vi "real_web_report.vi"(11 "httpRequestID":u32) -> (3 "httpRequestID out":u32)   [LabVIEW 2011]
uses:
  <vilib>/addons/database/Connection.llb/DB Tools Open Connec (String).vi
  databasePath.vi
  <vilib>/addons/database/Connection.llb/Conn Execute.vi
  <vilib>/addons/database/Recordset.llb/Rec Fetch Recordset Data (R).vi
  <vilib>/addons/database/Recordset.llb/Rec Destroy - Connection.vi
  <vilib>/addons/database/NI_Database_API.lvlib
  <vilib>/wsapi/NI_WebServices.lvlib
panel:
  out "error out":errorcluster
  out "error out 2":errorcluster
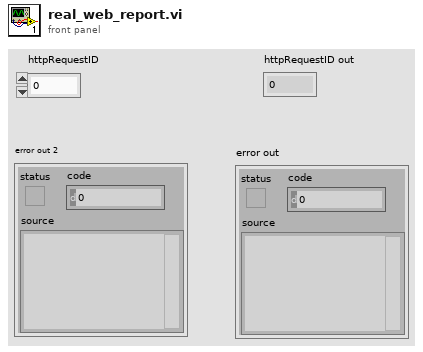
[diagram p1: front panel]
types:
  T1 = typedef "NI_Database_API.lvlib/Conn ObjectReference.ctl" = refnum<k1>
  T2 = typedef "NI_Database_API.lvlib/Rec ObjectReference.ctl" = refnum<k1>
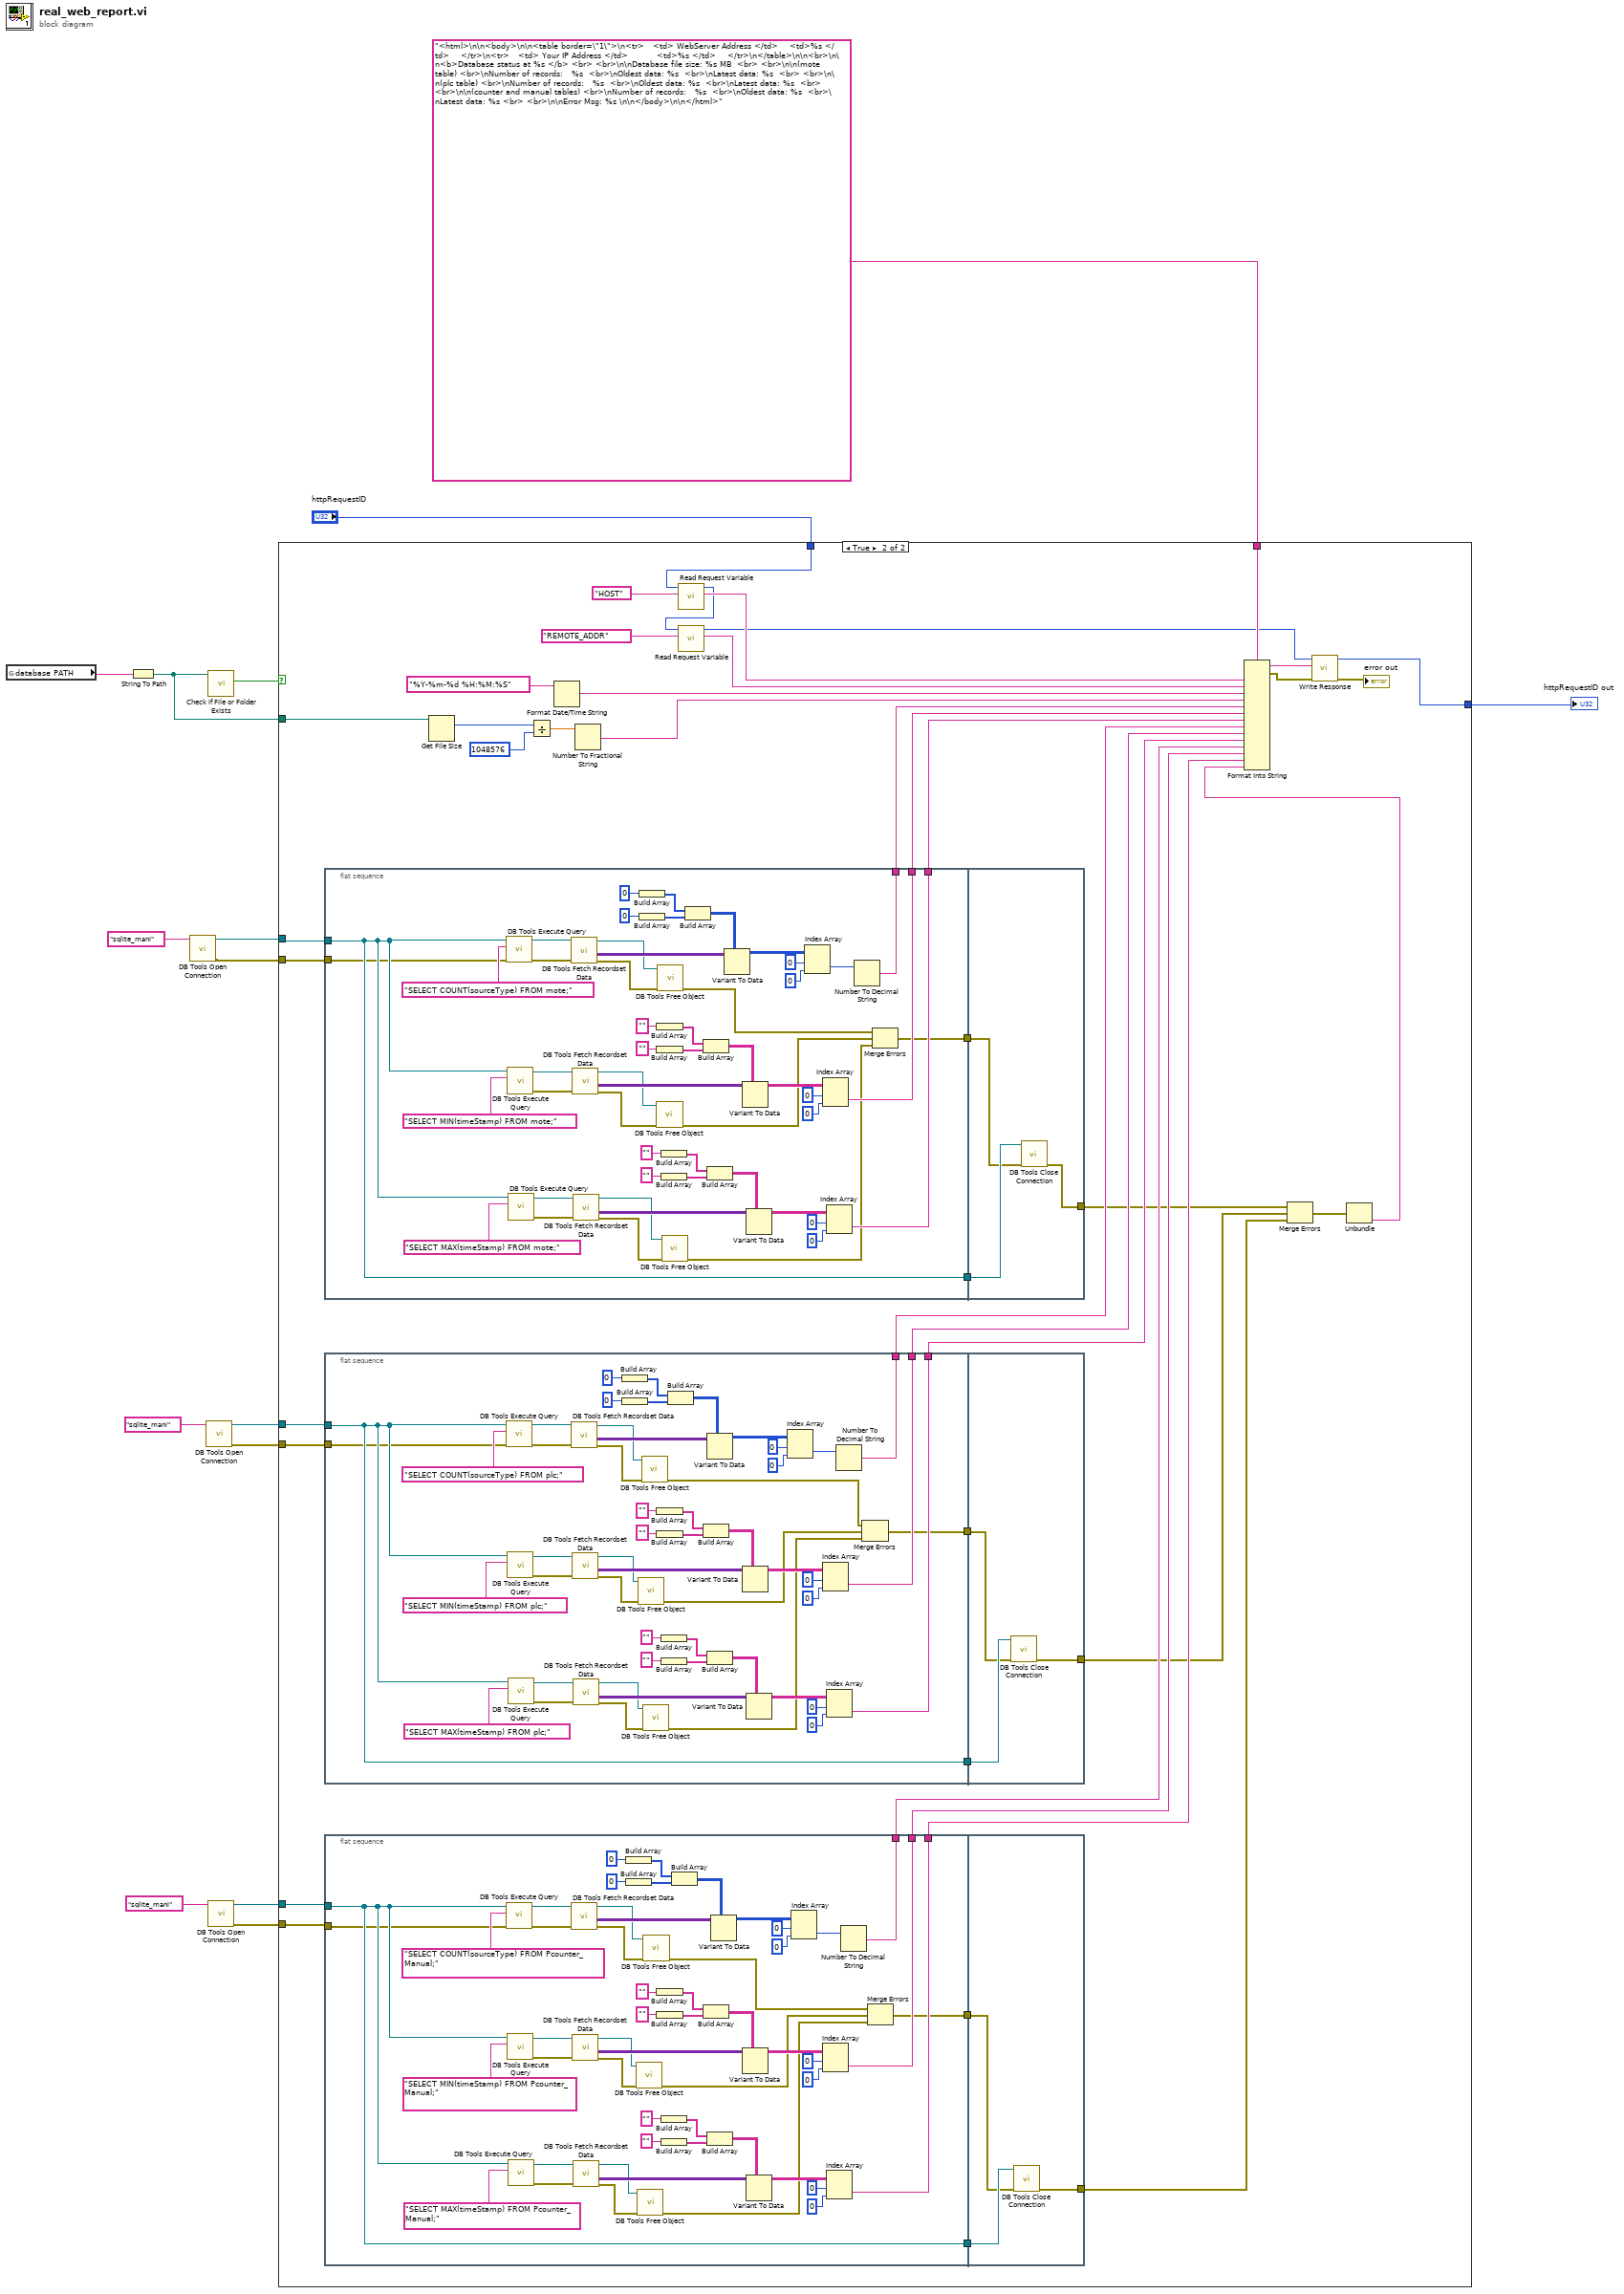
[diagram p0: block diagram]
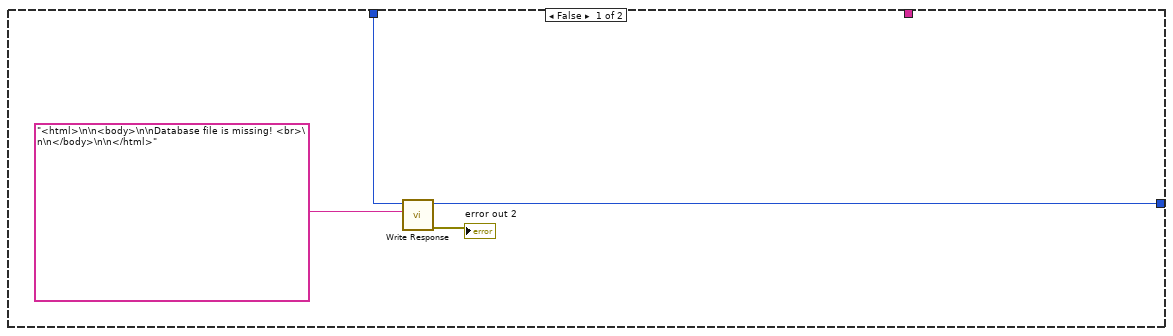
[diagram p2: hidden frame]
diagram:
  n1 = global read "databasePath.vi" "database PATH"() -> (w14:string)
  n2 = String To Path(string=w14) -> (path=w13:path)
  n3 = call-poly <vilib>:"DB Tools Open Connection.vi"("connection information"="sqlite_mani") -> ("error out"=w8:errorcluster, "connection reference"=w9:T1)  [unwired: 7 in]
  n4 = call-poly <vilib>:"DB Tools Open Connection.vi"("connection information"="sqlite_mani") -> ("error out"=w3:errorcluster, "connection reference"=w4:T1)  [unwired: 7 in]
  n5 = call <vilib>:"Check if File or Folder Exists.vi"("path"=w13) -> ("file or folder exists?"=w15:bool)  [unwired: 8 in, 2 out]
  n6 = call-poly <vilib>:"DB Tools Open Connection.vi"("connection information"="sqlite_mani") -> ("error out"=w1:errorcluster, "connection reference"=w2:T1)  [unwired: 7 in]
  n7 = case shown="True" w15 {
    tunnel: "httpRequestID" -> [w17 w46]
    tunnel: w13 -> [_ w60]
    tunnel: "<html>\n\n<body>\n\n<table border=\"1\">\n<tr>   <td> WebServer Address </td>    <td>%s </td>    </tr>\n<tr>   <td> Your IP Address </td>          <td>%s </td>    </tr>\n</table>\n\n<br>\n\n<b>Database status at %s </b> <br> <br>\n\nDatabase file size: %s MB  <br> <br>\n\n(mote table) <br>\nNumber of records:   %s  <br>\nOldest data: %s  <br>\nLatest data: %s  <br> <br>\n\n(plc table) <br>\nNumber of records:   %s  <br>\nOldest data: %s  <br>\nLatest data: %s  <br> <br>\n\n(counter and manual tables) <br>\nNumber of records:   %s  <br>\nOldest data: %s  <br>\nLatest data: %s <br> <br>\n\nError Msg: %s \n\n</body>\n\n</html>" -> [_ w56]
    tunnel: [w16 w53] -> w11
    tunnel: w9 -> [_ w40]
    tunnel: w8 -> [_ w39]
    tunnel: w4 -> [_ w34]
    tunnel: w3 -> [_ w33]
    tunnel: w2 -> [_ w32]
    tunnel: w1 -> [_ w31]
    frame False {
      n8 = call <vilib>:"Write Response.vi"("response string"="<html>\n\n<body>\n\nDatabase file is missing! <br>\n\n</body>\n\n</html>", "httpRequestID"=w17) -> ("error out"=→"error out 2":errorcluster, "httpRequestID out"=w16:u32)  [unwired: 1 in, 7 out]
    }
    frame True {
      n9 = flat-sequence {
        tunnel: [w213] -> w57
        tunnel: [w197] -> w44
        tunnel: [w187] -> w43
        tunnel: [w175] -> w42
        tunnel: [w186] -> w41
        tunnel: w40 -> [w186]
        tunnel: w39 -> [w185]
        tunnel: w42 -> [w228]
        tunnel: w41 -> [w229]
        tunnel: [w227] -> w24
        frame #0 {
          n10 = call-poly <vilib>:"DB Tools Execute Query.vi"("error in (no error)"=w185, "SQL query"="SELECT COUNT(sourceType) FROM mote;", "connection reference"=w186) -> ("error out"=w217:errorcluster, "recordset reference"=w216:T2)  [unwired: 5 in]
          n11 = call-poly <vilib>:"DB Tools Execute Query.vi"("SQL query"="SELECT MIN(timeStamp) FROM mote;", "connection reference"=w186) -> ("error out"=w212:errorcluster, "recordset reference"=w208:T2)  [unwired: 6 in]
          n12 = call-poly <vilib>:"DB Tools Execute Query.vi"("SQL query"="SELECT MAX(timeStamp) FROM mote;", "connection reference"=w186) -> ("error out"=w211:errorcluster, "recordset reference"=w207:T2)  [unwired: 6 in]
          n13 = call-poly <vilib>:"DB Tools Fetch Recordset Data.vi"("error in (no error)"=w217, "recordset reference"=w216) -> ("error out"=w184:errorcluster, "recordset data"=w222:variant[][], "recordset reference out"=w183:T2)  [unwired: 3 in]
          n14 = call-poly <vilib>:"DB Tools Fetch Recordset Data.vi"("error in (no error)"=w212, "recordset reference"=w208) -> ("error out"=w182:errorcluster, "recordset data"=w198:variant[][], "recordset reference out"=w181:T2)  [unwired: 3 in]
          n15 = call-poly <vilib>:"DB Tools Fetch Recordset Data.vi"("error in (no error)"=w211, "recordset reference"=w207) -> ("error out"=w180:errorcluster, "recordset data"=w188:variant[][], "recordset reference out"=w179:T2)  [unwired: 3 in]
          n16 = Build Array(i64 0) -> (w219:i64[])
          n17 = Build Array(i64 0) -> (w220:i64[])
          n18 = Build Array("") -> (w205:string[])
          n19 = Build Array("") -> (w204:string[])
          n20 = call-poly <vilib>:"DB Tools Free Object.vi"("error in (no error)"=w182, "recordset reference"=w181) -> ("error out"=w177:errorcluster)  [unwired: 8 in, 1 out]
          n21 = call-poly <vilib>:"DB Tools Free Object.vi"("error in (no error)"=w184, "recordset reference"=w183) -> ("error out"=w178:errorcluster)  [unwired: 8 in, 1 out]
          n22 = Build Array("") -> (w190:string[])
          n23 = Build Array("") -> (w191:string[])
          n24 = call-poly <vilib>:"DB Tools Free Object.vi"("error in (no error)"=w180, "recordset reference"=w179) -> ("error out"=w176:errorcluster)  [unwired: 8 in, 1 out]
          n25 = Build Array(w219, w220) -> (w223:i64[][])
          n26 = Build Array(w205, w204) -> (w202:string[][])
          n27 = Build Array(w190, w191) -> (w193:string[][])
          n28 = Variant To Data(type=w223, Variant=w222) -> (data=w224:i64[][])  [unwired: 1 in, 1 out]
          n29 = Variant To Data(type=w202, Variant=w198) -> (data=w201:string[][])  [unwired: 1 in, 1 out]
          n30 = Variant To Data(type=w193, Variant=w188) -> (data=w194:string[][])  [unwired: 1 in, 1 out]
          n31 = Index Array(array=w224, index (row)=0, index (col)=0 ("disabled index (col)")) -> (element=w215:i64)
          n32 = Index Array(array=w201, index (row)=0, index (col)=0 ("disabled index (col)")) -> (element=w197:string)
          n33 = Index Array(array=w194, index (row)=0, index (col)=0 ("disabled index (col)")) -> (element=w187:string)
          n34 = Number To Decimal String(number=w215) -> (decimal integer string=w213:string)  [unwired: 1 in]
          n35 = Merge Errors(w178, w177, w176) -> (w175:errorcluster)
        }
        frame #1 {
          n36 = call <vilib>:"DB Tools Close Connection.vi"("error in (no error)"=w228, "connection reference"=w229) -> ("error out"=w227:errorcluster)  [unwired: 5 in]
        }
      }
      n37 = flat-sequence {
        tunnel: [w158] -> w30
        tunnel: [w142] -> w29
        tunnel: [w132] -> w28
        tunnel: [w120] -> w38
        tunnel: [w131] -> w37
        tunnel: w34 -> [w131]
        tunnel: w33 -> [w130]
        tunnel: w38 -> [w173]
        tunnel: w37 -> [w174]
        tunnel: [w172] -> w23
        frame #0 {
          n38 = call-poly <vilib>:"DB Tools Execute Query.vi"("error in (no error)"=w130, "SQL query"="SELECT COUNT(sourceType) FROM plc;", "connection reference"=w131) -> ("error out"=w162:errorcluster, "recordset reference"=w161:T2)  [unwired: 5 in]
          n39 = call-poly <vilib>:"DB Tools Execute Query.vi"("SQL query"="SELECT MIN(timeStamp) FROM plc;", "connection reference"=w131) -> ("error out"=w157:errorcluster, "recordset reference"=w153:T2)  [unwired: 6 in]
          n40 = call-poly <vilib>:"DB Tools Execute Query.vi"("SQL query"="SELECT MAX(timeStamp) FROM plc;", "connection reference"=w131) -> ("error out"=w156:errorcluster, "recordset reference"=w152:T2)  [unwired: 6 in]
          n41 = call-poly <vilib>:"DB Tools Fetch Recordset Data.vi"("error in (no error)"=w162, "recordset reference"=w161) -> ("error out"=w129:errorcluster, "recordset data"=w167:variant[][], "recordset reference out"=w128:T2)  [unwired: 3 in]
          n42 = call-poly <vilib>:"DB Tools Fetch Recordset Data.vi"("error in (no error)"=w157, "recordset reference"=w153) -> ("error out"=w127:errorcluster, "recordset data"=w143:variant[][], "recordset reference out"=w125:T2)  [unwired: 3 in]
          n43 = call-poly <vilib>:"DB Tools Fetch Recordset Data.vi"("error in (no error)"=w156, "recordset reference"=w152) -> ("error out"=w126:errorcluster, "recordset data"=w133:variant[][], "recordset reference out"=w124:T2)  [unwired: 3 in]
          n44 = Build Array(i64 0) -> (w164:i64[])
          n45 = Build Array(i64 0) -> (w165:i64[])
          n46 = call-poly <vilib>:"DB Tools Free Object.vi"("error in (no error)"=w127, "recordset reference"=w125) -> ("error out"=w122:errorcluster)  [unwired: 8 in, 1 out]
          n47 = call-poly <vilib>:"DB Tools Free Object.vi"("error in (no error)"=w129, "recordset reference"=w128) -> ("error out"=w123:errorcluster)  [unwired: 8 in, 1 out]
          n48 = call-poly <vilib>:"DB Tools Free Object.vi"("error in (no error)"=w126, "recordset reference"=w124) -> ("error out"=w121:errorcluster)  [unwired: 8 in, 1 out]
          n49 = Build Array("") -> (w150:string[])
          n50 = Build Array("") -> (w149:string[])
          n51 = Build Array("") -> (w135:string[])
          n52 = Build Array("") -> (w136:string[])
          n53 = Build Array(w164, w165) -> (w168:i64[][])
          n54 = Build Array(w150, w149) -> (w147:string[][])
          n55 = Variant To Data(type=w168, Variant=w167) -> (data=w169:i64[][])  [unwired: 1 in, 1 out]
          n56 = Build Array(w135, w136) -> (w138:string[][])
          n57 = Variant To Data(type=w147, Variant=w143) -> (data=w146:string[][])  [unwired: 1 in, 1 out]
          n58 = Variant To Data(type=w138, Variant=w133) -> (data=w139:string[][])  [unwired: 1 in, 1 out]
          n59 = Index Array(array=w169, index (row)=0, index (col)=0 ("disabled index (col)")) -> (element=w160:i64)
          n60 = Index Array(array=w146, index (row)=0, index (col)=0 ("disabled index (col)")) -> (element=w142:string)
          n61 = Index Array(array=w139, index (row)=0, index (col)=0 ("disabled index (col)")) -> (element=w132:string)
          n62 = Number To Decimal String(number=w160) -> (decimal integer string=w158:string)  [unwired: 1 in]
          n63 = Merge Errors(w123, w122, w121) -> (w120:errorcluster)
        }
        frame #1 {
          n64 = call <vilib>:"DB Tools Close Connection.vi"("error in (no error)"=w173, "connection reference"=w174) -> ("error out"=w172:errorcluster)  [unwired: 5 in]
        }
      }
      n65 = flat-sequence {
        tunnel: [w103] -> w27
        tunnel: [w87] -> w26
        tunnel: [w77] -> w25
        tunnel: [w65] -> w36
        tunnel: [w76] -> w35
        tunnel: w32 -> [w76]
        tunnel: w31 -> [w75]
        tunnel: w36 -> [w118]
        tunnel: w35 -> [w119]
        tunnel: [w117] -> w22
        frame #0 {
          n66 = call-poly <vilib>:"DB Tools Execute Query.vi"("error in (no error)"=w75, "SQL query"="SELECT COUNT(sourceType) FROM Pcounter_Manual;", "connection reference"=w76) -> ("error out"=w107:errorcluster, "recordset reference"=w106:T2)  [unwired: 5 in]
          n67 = call-poly <vilib>:"DB Tools Execute Query.vi"("SQL query"="SELECT MIN(timeStamp) FROM Pcounter_Manual;", "connection reference"=w76) -> ("error out"=w102:errorcluster, "recordset reference"=w98:T2)  [unwired: 6 in]
          n68 = call-poly <vilib>:"DB Tools Execute Query.vi"("SQL query"="SELECT MAX(timeStamp) FROM Pcounter_Manual;", "connection reference"=w76) -> ("error out"=w101:errorcluster, "recordset reference"=w97:T2)  [unwired: 6 in]
          n69 = call-poly <vilib>:"DB Tools Fetch Recordset Data.vi"("error in (no error)"=w107, "recordset reference"=w106) -> ("error out"=w74:errorcluster, "recordset data"=w112:variant[][], "recordset reference out"=w73:T2)  [unwired: 3 in]
          n70 = call-poly <vilib>:"DB Tools Fetch Recordset Data.vi"("error in (no error)"=w102, "recordset reference"=w98) -> ("error out"=w72:errorcluster, "recordset data"=w88:variant[][], "recordset reference out"=w71:T2)  [unwired: 3 in]
          n71 = call-poly <vilib>:"DB Tools Fetch Recordset Data.vi"("error in (no error)"=w101, "recordset reference"=w97) -> ("error out"=w70:errorcluster, "recordset data"=w78:variant[][], "recordset reference out"=w69:T2)  [unwired: 3 in]
          n72 = Build Array(i64 0) -> (w109:i64[])
          n73 = Build Array(i64 0) -> (w110:i64[])
          n74 = call-poly <vilib>:"DB Tools Free Object.vi"("error in (no error)"=w72, "recordset reference"=w71) -> ("error out"=w67:errorcluster)  [unwired: 8 in, 1 out]
          n75 = call-poly <vilib>:"DB Tools Free Object.vi"("error in (no error)"=w70, "recordset reference"=w69) -> ("error out"=w66:errorcluster)  [unwired: 8 in, 1 out]
          n76 = call-poly <vilib>:"DB Tools Free Object.vi"("error in (no error)"=w74, "recordset reference"=w73) -> ("error out"=w68:errorcluster)  [unwired: 8 in, 1 out]
          n77 = Build Array("") -> (w95:string[])
          n78 = Build Array("") -> (w94:string[])
          n79 = Build Array("") -> (w80:string[])
          n80 = Build Array("") -> (w81:string[])
          n81 = Build Array(w109, w110) -> (w113:i64[][])
          n82 = Build Array(w95, w94) -> (w92:string[][])
          n83 = Build Array(w80, w81) -> (w83:string[][])
          n84 = Variant To Data(type=w113, Variant=w112) -> (data=w114:i64[][])  [unwired: 1 in, 1 out]
          n85 = Variant To Data(type=w92, Variant=w88) -> (data=w91:string[][])  [unwired: 1 in, 1 out]
          n86 = Variant To Data(type=w83, Variant=w78) -> (data=w84:string[][])  [unwired: 1 in, 1 out]
          n87 = Index Array(array=w114, index (row)=0, index (col)=0 ("disabled index (col)")) -> (element=w105:i64)
          n88 = Index Array(array=w91, index (row)=0, index (col)=0 ("disabled index (col)")) -> (element=w87:string)
          n89 = Index Array(array=w84, index (row)=0, index (col)=0 ("disabled index (col)")) -> (element=w77:string)
          n90 = Number To Decimal String(number=w105) -> (decimal integer string=w103:string)  [unwired: 1 in]
          n91 = Merge Errors(w68, w67, w66) -> (w65:errorcluster)
        }
        frame #1 {
          n92 = call <vilib>:"DB Tools Close Connection.vi"("error in (no error)"=w118, "connection reference"=w119) -> ("error out"=w117:errorcluster)  [unwired: 5 in]
        }
      }
      n93 = Get File Size(file=w60) -> (size (in bytes)=w61:i64)  [unwired: 1 in, 2 out]
      n94 = Divide(x=w61, y=i64 1048576) -> (x/y=w62:dbl)
      n95 = Format Date/Time String(time format string (%c)="%Y-%m-%d %H:%M:%S") -> (date/time string=w59:string)  [unwired: 2 in]
      n96 = Number To Fractional String(number=w62) -> (F-format string=w58:string)  [unwired: 3 in]
      n97 = call <vilib>:"Read Request Variable.vi"("variable name"="HOST", "httpRequestID"=w46) -> ("value"=w49:string, "httpRequestID out"=w47:u32)  [unwired: 7 in, 1 out]
      n98 = call <vilib>:"Read Request Variable.vi"("variable name"="REMOTE_ADDR", "httpRequestID"=w47) -> ("value"=w48:string, "httpRequestID out"=w45:u32)  [unwired: 7 in, 1 out]
      n99 = Merge Errors(w24, w23, w22) -> (w21:errorcluster)
      n100 = Unbundle(w21) -> ("source"=w20:string)  [unwired: 2 out]
      n101 = Format Into String(format string=w56, w49, w48, w59, w58, w57, w44, w43, w30, w29, w28, w27, w26, w25, w20) -> (resulting string=w54:string, error out=w52:errorcluster)  [unwired: 2 in]
      n102 = call <vilib>:"Write Response.vi"("error in (no error)"=w52, "response string"=w54, "httpRequestID"=w45) -> ("error out"=→"error out":errorcluster, "httpRequestID out"=w53:u32)  [unwired: 7 out]
    }
  }
  "httpRequestID out" <- w11
